vi "Read Measurement Function Ring.vi"(8 "error in (no error)":errorcluster, 11 "Generic Digital Multi Meter in":refnum<class "Generic Digital Multi Meter.lvclass">) -> (0 "error out":errorcluster, 2 "Strings And Values []":T1, 3 "Generic Digital Multi Meter out":refnum<class "Generic Digital Multi Meter.lvclass">)   [LabVIEW 2014, in "Generic Digital Multi Meter.lvlib" / "Generic Digital Multi Meter.lvclass"]
uses:
  Generic Digital Multi Meter.lvclass
  <vilib>/Utility/miscctls.llb/LVStringsAndValuesArrayTypeDef_U16.ctl
  Generic Digital Multi Meter.lvclass/Generic Digital Multi Meter.ctl
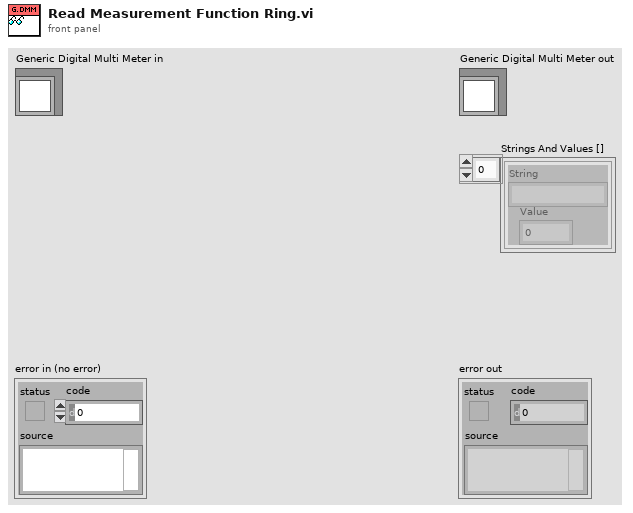
[diagram p1: front panel]
types:
  T1 = typedef "LVStringsAndValuesArrayTypeDef_U16.ctl" = cluster{"String":string, "Value":u16}[]
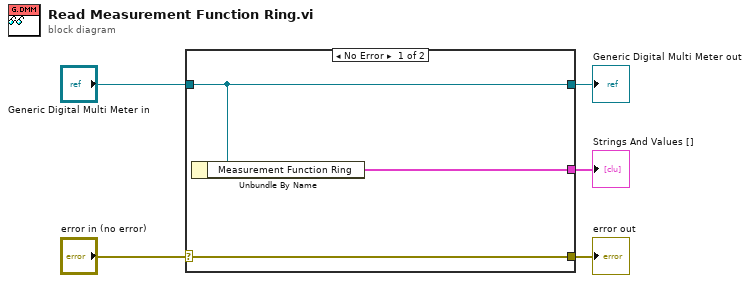
[diagram p0: block diagram]
diagram:
  n1 = case shown="No Error" "error in (no error)" {
    selector: "error in (no error)" -> [w8 w9]
    tunnel: [w8 w9] -> w4
    tunnel: [w7 w10] -> w2
    tunnel: "Generic Digital Multi Meter in" -> [w7 w10]
    tunnel: [w6 _] -> w1
    frame No Error {
      n2 = Unbundle By Name(w7) -> ("Measurement Function Ring"=w6:T1)
    }
    frame Error {
    }
  }
  "error out" <- w4
  "Generic Digital Multi Meter out" <- w2
  "Strings And Values []" <- w1
